vi "CopyCrossCorrelationResult.vi"(0 "tracker":u64) -> (1 "tracker":u64, 2 "resultArray":sgl[](array[numeric]))   [LabVIEW 2011]
uses:
  CpuTrackDLL.vi
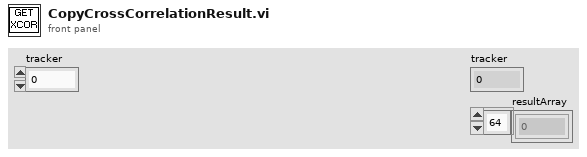
[diagram p1: front panel]
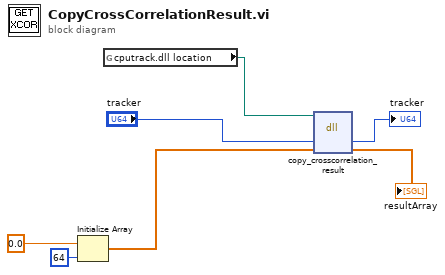
[diagram p0: block diagram]
diagram:
  n1 = Initialize Array(sgl 0.0 ("element"), 64 ("dimension size")) -> (w1:sgl[])
  n2 = global read "CpuTrackDLL.vi" "cputrack.dll location"() -> (w7:path)
  n3 = dll-call lib="?" fn="copy_crosscorrelation_result"(path in=w7, "tracker"="tracker", "resultArray"=w1) -> ("tracker"=→"tracker":u64, "resultArray"=→"resultArray":sgl[])  [unwired: 3 in, 2 out]
